vi "Low_Pass_Filter1.vi"(1 "Tf":dbl, 2 "Ts":dbl, 3 "yk":dbl) -> (0 "señal filtrada":dbl)   [LabVIEW 2021]
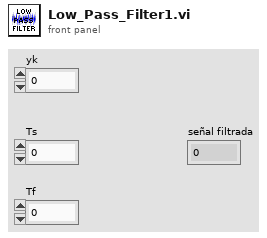
[diagram p1: front panel]
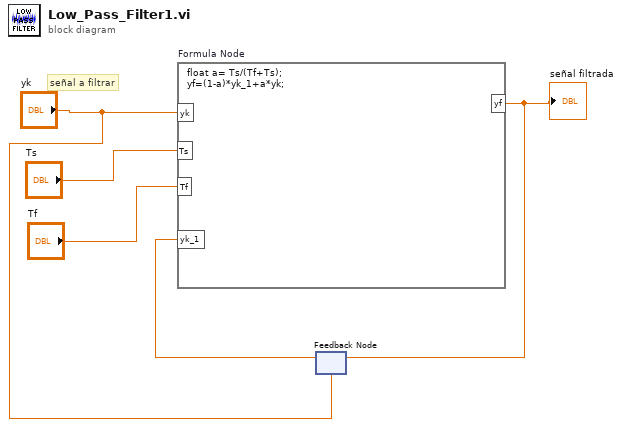
[diagram p0: block diagram]
diagram:
  # "señal a filtrar"
  n1 = feedback #1("yk") -> (w2:dbl)
  n2 = formula code="float a= Ts/(Tf+Ts);\nyf=(1-a)*yk_1+a*yk;"("yk"="yk", "Ts"="Ts", "Tf"="Tf", "yk_1"=w2) -> ("yf"=w3:dbl)
  "señal filtrada" <- w3
  n3 = feedback-in #1(w3) -> ()
